vi "inclinePIP.vi"(8 "error in (no error)":errorcluster, 10 "QUICK_KEYS":bool, 11 "INCLINE":bool) -> (0 "error out":errorcluster, 3 "INCLINE-14":string)   [LabVIEW 2018]
uses:
  Global_1259.vi
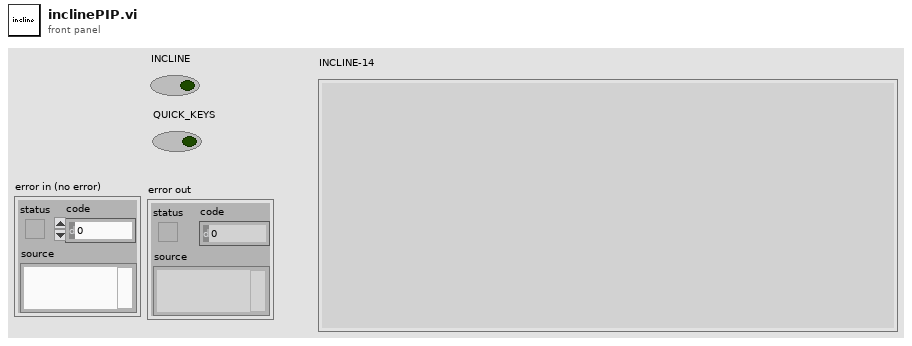
[diagram p1: front panel]
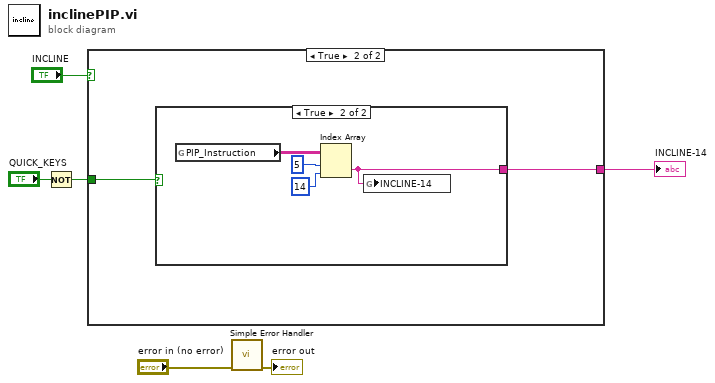
[diagram p0: block diagram]
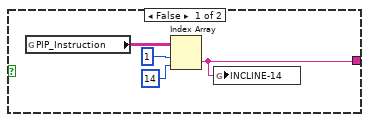
[diagram p3: hidden frame]
diagram:
  n1 = Not(x="QUICK_KEYS") -> (.not. x?=w1:bool)
  n2 = case shown="True" "INCLINE" {
    tunnel: [_ w8] -> w6
    tunnel: w1 -> [_ w7]
    frame False {
    }
    frame True {
      n3 = case shown="True" w7 {
        tunnel: [w9 w13] -> w8
        frame False {
          n4 = global read "Global_1259.vi" "PIP_Instruction"() -> (w12:string[][])
          n5 = Index Array(array=w12, index (row)=1, index (col)=14 ("disabled index (col)")) -> (element=w9:string)
          n6 = global write "Global_1259.vi" "INCLINE-14"(w9) -> ()
        }
        frame True {
          n7 = global read "Global_1259.vi" "PIP_Instruction"() -> (w16:string[][])
          n8 = Index Array(array=w16, index (row)=5, index (col)=14 ("disabled index (col)")) -> (element=w13:string)
          n9 = global write "Global_1259.vi" "INCLINE-14"(w13) -> ()
        }
      }
    }
  }
  "INCLINE-14" <- w6
  n10 = call <vilib>:"Simple Error Handler.vi"("error in (no error)"="error in (no error)") -> ("error out"=→"error out":errorcluster)  [unwired: 4 in, 4 out]
